vi "Temperature monitoring system.vi"() -> ()   [LabVIEW 2012]
panel:
  out "result":dbl
  in  "stop":bool
  out "30<avg<60":bool
  out "<30":bool
  out ">60":bool
  in  "Current":dbl(slide) scale=0.0..100.0
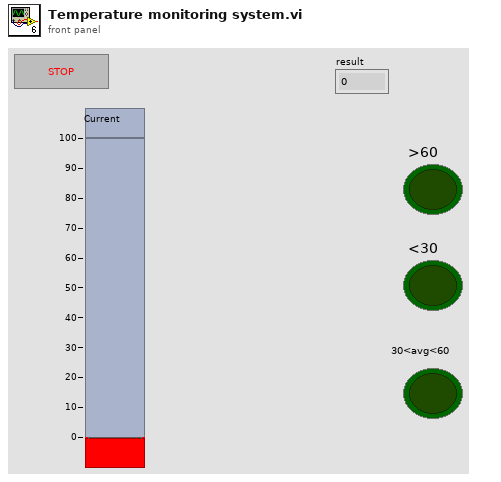
[diagram p1: front panel]
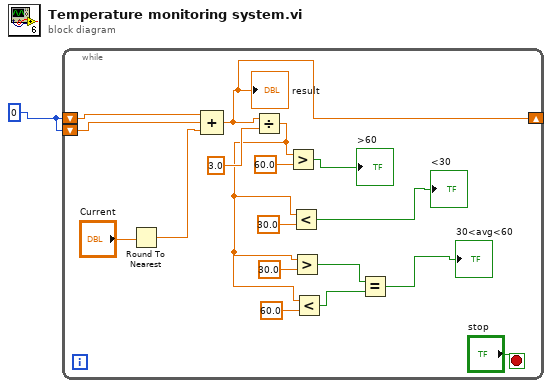
[diagram p0: block diagram]
diagram:
  w1 = 0
  n1 = while {
    shift-right: [w2] -> _
    shift-left: w1 -> [w13]
    shift-left: w1 -> [w12]
    stop <- "stop" stop-if-true
    n2 = Round To Nearest(number="Current") -> (nearest integer value=w10:dbl)
    n3 = Compound Arithmetic op=ADD(w13, w12, w10) -> (w2:dbl)
    "result" <- w2
    n4 = Divide(x=w2, y=3.0) -> (x/y=w3:dbl)
    n5 = Greater?(x=w3, y=60.0) -> (0:→">60":bool)
    n6 = Less?(x=w3, y=30.0) -> (x < y?=→"<30":bool)
    n7 = Greater?(x=w3, y=30.0) -> (0:w16:bool)
    n8 = Less?(x=w3, y=60.0) -> (x < y?=w15:bool)
    n9 = Equal?(x=w16, y=w15) -> (x = y?=→"30<avg<60":bool)
  }
